vi "Set Color.vi"(8 "error in (no error)":errorcluster, 10 "Color Message.lvclass":refnum<class "Color Message.lvclass">, 11 "[V]System Tree View in":refnum<class "[V]System Tree View.lvclass">) -> (0 "error out":errorcluster, 3 "[V]System Tree View out":refnum<class "[V]System Tree View.lvclass">)   [LabVIEW 2020, in "[V]System Tree View.lvlib" / "[V]System Tree View.lvclass"]
uses:
  [V]System Tree View.lvclass
  Color Interface/Color/Color Message.lvclass
  Color Interface/Color/Color Message.lvclass/Color Message.ctl
  Depden On/Abstruct View/Abstruct View/Abstruct View.lvclass/Abstruct View.ctl
  Depden On/Abstruct View/Abstruct View/Data Accessors/Read Core VI.vi
  Color Interface/Color/Accessors/Read BG Color.vi
  Color Interface/Color/Accessors/Read Fornt Color.vi
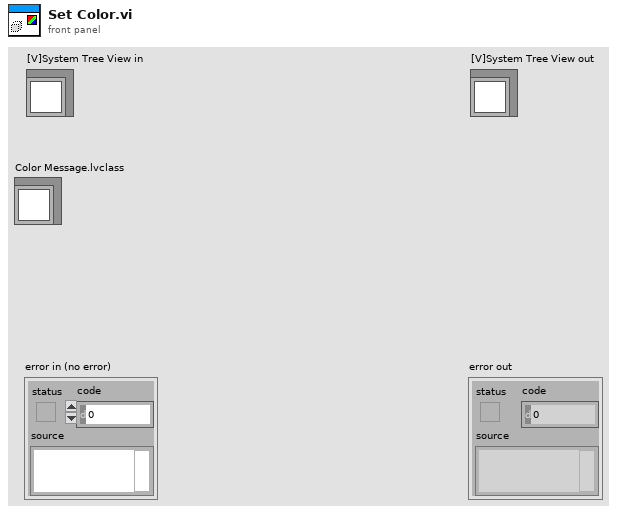
[diagram p1: front panel]
types:
  T1 = cluster{"Bold":bool, "Justification":enum16{"Left", "Center", "Right"}, "Font:Size":u32, "Font:Color":u32, "BG Color":u32}
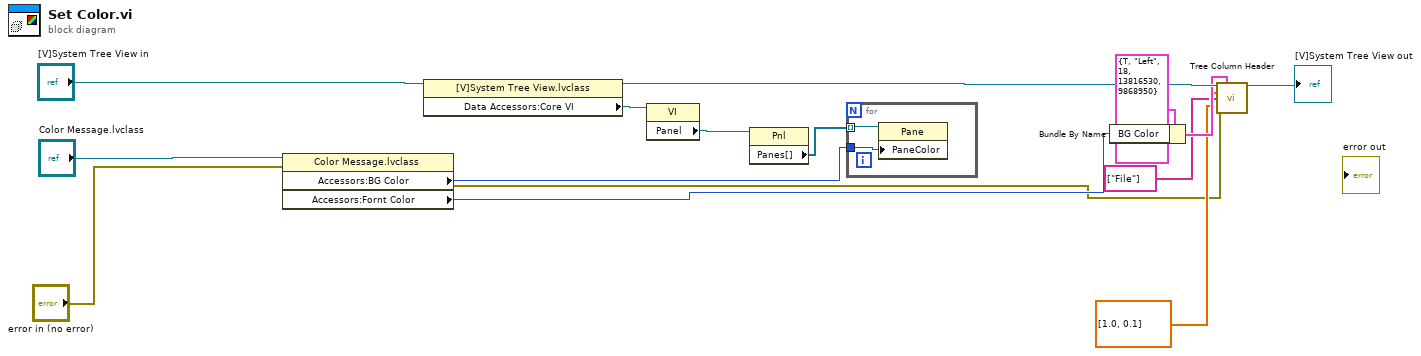
[diagram p0: block diagram]
diagram:
  n1 = property class="Color Message.lvclass"(reference="Color Message.lvclass", error in="error in (no error)") -> (error out=w5:errorcluster, "Accessors:BG Color"=w1:u32, "Accessors:Fornt Color"=w11:u32)  [unwired: 1 out]
  n2 = property class="[V]System Tree View.lvclass"(reference="[V]System Tree View in") -> (reference out=w10:refnum<class "[V]System Tree View.lvclass">, "Data Accessors:Core VI"=w4:refnum<vi>)  [unwired: 1 in, 1 out]
  n3 = property class="VI"(reference=w4) -> ("Panel"=w3:refnum<vi>)  [unwired: 1 in, 2 out]
  n4 = property class="Pnl"(reference=w3) -> ("Panes[]"=w2:refnum<vi>[])  [unwired: 1 in, 2 out]
  n5 = for {
    tunnel: w2 -> [w17] mode=indexing
    tunnel: w1 -> [w16]
    n6 = property class="Pane"(reference=w17, "PaneColor"=w16) -> ()  [unwired: 1 in, 2 out]
  }
  n7 = Bundle By Name(cluster=T1 {"Bold"=TRUE, "Justification"=enum."Left", "Font:Size"=18, "Font:Color"=13816530, "BG Color"=9868950} ("Style"), "BG Color"=w11) -> (w8:T1)
  n8 = call "Tree Column Header.vi"("[V]System Tree View in"=w10, "Style"=w8, "Header Width Ratio"=dbl[] [1.0, 0.1], "Header Names"=string[] ["File"], "error in (no error)"=w5) -> ("[V]System Tree View out"=→"[V]System Tree View out":refnum<class "[V]System Tree View.lvclass">)  [unwired: 9 in, 1 out]
